vi "Traffic_Light_System.vi"() -> ()   [LabVIEW 2020]
panel:
  in  "stop":bool
  in  "NUMBER OF BLINKS":i32=4
  in  "YELLOW BLINK TIME":u32=500
  in  "GREEN BLINK TIME":u32=1000
  in  "RED BLINK TIME":u32=3000
  out "GREEN":bool
  out "YELLOW":bool
  out "RED":bool
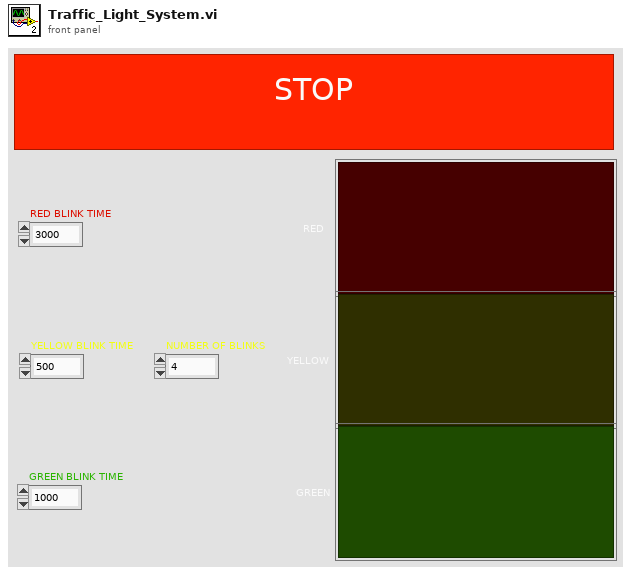
[diagram p1: front panel]
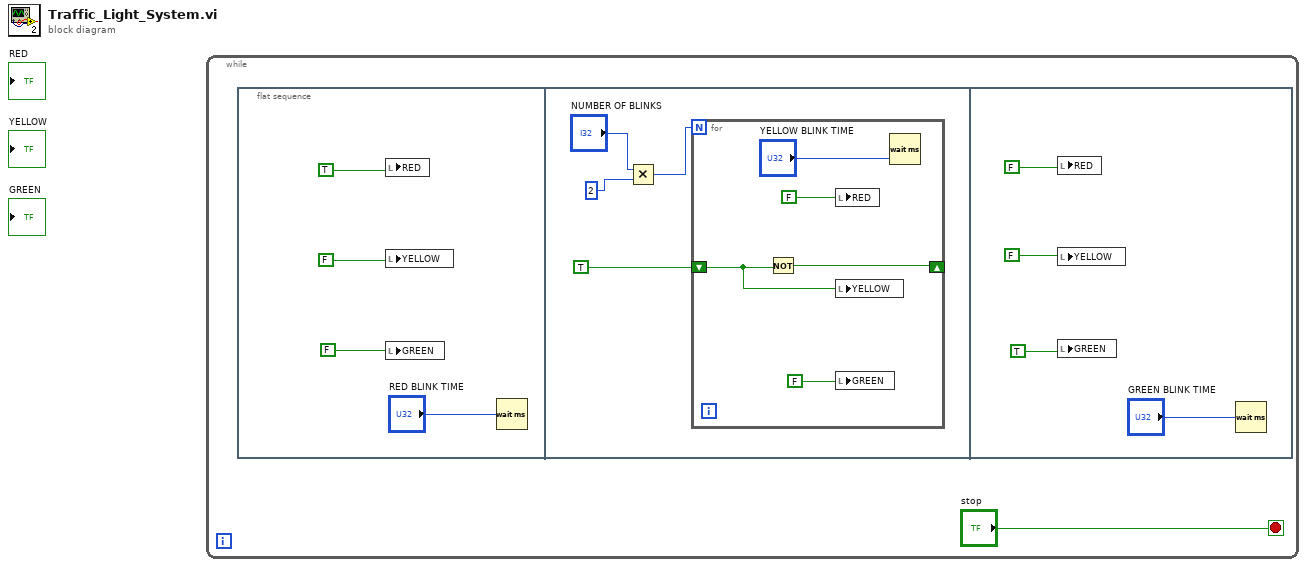
[diagram p0: block diagram]
diagram:
  n1 = while {
    stop <- "stop" stop-if-true
    n2 = flat-sequence {
      frame #0 {
        n3 = local write "RED"(TRUE) -> ()
        n4 = local write "YELLOW"(FALSE) -> ()
        n5 = local write "GREEN"(FALSE) -> ()
        n6 = Wait (ms)(milliseconds to wait="RED BLINK TIME") -> ()  [unwired: 1 out]
      }
      frame #1 {
        n7 = Multiply(x="NUMBER OF BLINKS", y=2) -> (x*y=w6:i32)
        n8 = for {
          N: w6 -> [_]
          shift-right: [w14] -> _
          shift-left: TRUE -> [w13]
          n9 = Not(x=w13) -> (.not. x?=w14:bool)
          n10 = local write "RED"(FALSE) -> ()
          n11 = local write "YELLOW"(w13) -> ()
          n12 = local write "GREEN"(FALSE) -> ()
          n13 = Wait (ms)(milliseconds to wait="YELLOW BLINK TIME") -> ()  [unwired: 1 out]
        }
      }
      frame #2 {
        n14 = local write "RED"(FALSE) -> ()
        n15 = local write "YELLOW"(FALSE) -> ()
        n16 = local write "GREEN"(TRUE) -> ()
        n17 = Wait (ms)(milliseconds to wait="GREEN BLINK TIME") -> ()  [unwired: 1 out]
      }
    }
  }
